vi "GetSwerveRawAzimuth.vi"(1 "Calibrate Wheels":bool, 2 "Azimuth Falcon Refnum":string="My Motor RefNum") -> (0 "Position (Raw Sensor Units)":dbl)   [LabVIEW 2023]
doc: "Gets the raw azimuth position from the non-absolute encoder on the Falcon. Handles motor controller and RoboRIO brownout scenarios. Re-zeroing the swerve modules also occurs here."
uses:
  GRNF_GenericMotor.vi
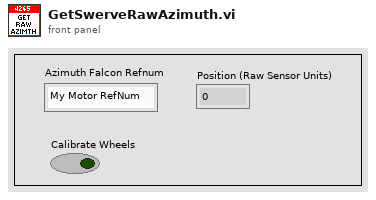
[diagram p1: front panel]
types:
  T1 = typedef "WPI_MotorControlDeviceRef.ctl" = cluster{"DeviceStatus":errorcluster, "Type":T2, "PWM":cluster{"PWM Channel":T3, "DeadBand":T4}, "CAN":cluster{"Device Number":u8, "SetOutput VI Ref":variant, "GetOutput VI Ref":variant, "Enable VI Ref":variant, "Disable VI Ref":variant, "Data":variant}, "Invert":bool, "DIO PWM":cluster{"PWM \"Enable\" Channel":T3, "DIOChannel":T5, "PWM Rate":dbl}}
  T2 = typedef "WPI_MotorControlType.ctl" = enum16{"PWM", "CAN", "DIO PWM"}
  T3 = typedef "FPGA_DIOPWMChannel.ctl" = enum8{"PWM 0", "PWM 1", "PWM 2", "PWM 3", "PWM 4", "PWM 5", "PWM 6", "PWM 7", "PWM 8", "PWM 9", "PWM MXP 0", "PWM MXP 1", "PWM MXP 2", "PWM MXP 3", "PWM MXP 4", "PWM MXP 5", "PWM MXP 6", "PWM MXP 7", "PWM MXP 8", "PWM MXP 9", "Invalid"}
  T4 = typedef "WPI_PWMDeadband.ctl" = cluster{"Name":string, "maxPositivePwm":i32, "minPositivePwm":i32, "centerPwm":i32, "maxNegativePwm":i32, "minNegativePwm":i32, "angularRange":u16}
  T5 = typedef "FPGA_DIOChannel.ctl" = enum8{"DIO 0", "DIO 1", "DIO 2", "DIO 3", "DIO 4", "DIO 5", "DIO 6", "DIO 7", "DIO 8", "DIO 9", "DIO MXP 0", "DIO MXP 1", "DIO MXP 2", "DIO MXP 3", "DIO MXP 4", "DIO MXP 5", "DIO MXP 6", "DIO MXP 7", "DIO MXP 8", "DIO MXP 9", "DIO MXP 10", "DIO MXP 11", "DIO MXP 12", "DIO MXP 13", "DIO MXP 14", "DIO MXP 15", "SPI Port CS1", "SPI Port CS2", "SPI Port CS3", "SPI Port MISO", "SPI Port MOSI", "Invalid"}
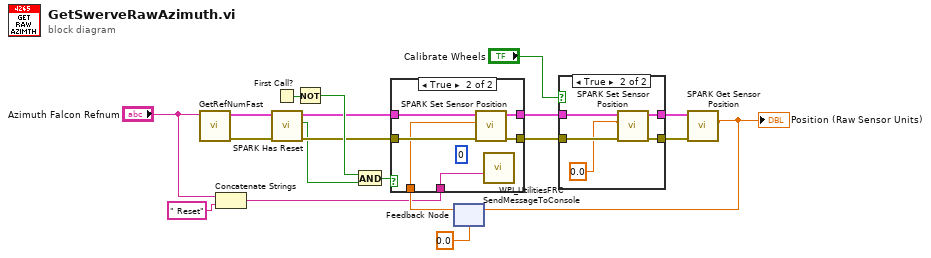
[diagram p0: block diagram]
diagram:
  n1 = call-poly "GetRefNumFast.vi"("RefNum Name"="Azimuth Falcon Refnum") -> ("Error"=w7:errorcluster, "Device Reference"=w8:T1)  [unwired: 5 in]
  n2 = Concatenate Strings("Azimuth Falcon Refnum", " Reset" ("string")) -> (w10:string)
  n3 = First Call?() -> (First Call?: T/F=w18:bool)
  n4 = call <vilib>:"SPARK Has Reset.vi"("error in (no error)"=w7, "MotorControlDevRef in"=w8) -> ("error out"=w5:errorcluster, "Has Reset?"=w4:bool, "MotorControlDevRef out"=w6:T1)  [unwired: 6 in, 1 out]
  n5 = Not(x=w18) -> (.not. x?=w19:bool)
  n6 = And(x=w19, y=w4) -> (x .and. y?=w17:bool)
  n7 = feedback #1(0.0 ("Position (Raw Sensor Units)")) -> (w14:dbl)
  n8 = case shown="True" w17 {
    tunnel: w5 -> [w20 w25]
    tunnel: w6 -> [w21 w26]
    tunnel: [w21 w23] -> w15
    tunnel: [w20 w22] -> w16
    tunnel: w14 -> [_ w24]
    tunnel: w10 -> [_ w27]
    frame False {
    }
    frame True {
      (unwired) u32 0 ("pidLoopIdx")
      n9 = call <vilib>:"SPARK Set Sensor Position.vi"("error in"=w25, "Position"=w24, "MotorControlDeviceRef"=w26) -> ("error out"=w22:errorcluster, "MotorControlDeviceRef"=w23:T1)  [unwired: 7 in]
      n10 = call <vilib>:"WPI_UtilitiesFRC SendMessageToConsole.vi"("Message"=w27) -> ()  [unwired: 14 in, 1 out]
    }
  }
  n11 = case shown="True" "Calibrate Wheels" {
    tunnel: w16 -> [w28 w31]
    tunnel: w15 -> [w29 w32]
    tunnel: [w29 w33] -> w3
    tunnel: [w28 w34] -> w2
    frame False {
    }
    frame True {
      n12 = call <vilib>:"SPARK Set Sensor Position.vi"("error in"=w31, "Position"=0.0 ("New Sensor Position"), "MotorControlDeviceRef"=w32) -> ("error out"=w34:errorcluster, "MotorControlDeviceRef"=w33:T1)  [unwired: 7 in]
    }
  }
  n13 = call <vilib>:"SPARK Get Sensor Position.vi"("error in (no error)"=w2, "MotorControlDevRef in"=w3) -> ("Sensor Position"=w1:dbl)  [unwired: 6 in, 3 out]
  "Position (Raw Sensor Units)" <- w1
  n14 = feedback-in #1(w1) -> ()
